vi "Command Select.vi"(8 "error in (no error)":errorcluster, 9 "Node Id":u8, 11 "Cmd Type":T1) -> (0 "error out":errorcluster, 2 "Cmd Str":string)   [LabVIEW 2011]
uses:
  Enumerator/CmdType.ctl
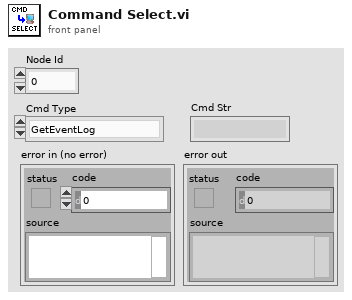
[diagram p1: front panel]
types:
  T1 = typedef "CmdType.ctl" = enum16{"GetEventLog", "DelTransaction", "InvalidMessage", "RelayControl", "RelayOff", "RelayOn", "VaildMessage", "EventPolling", "StoppingWaiting", "PromptKeying-in"}
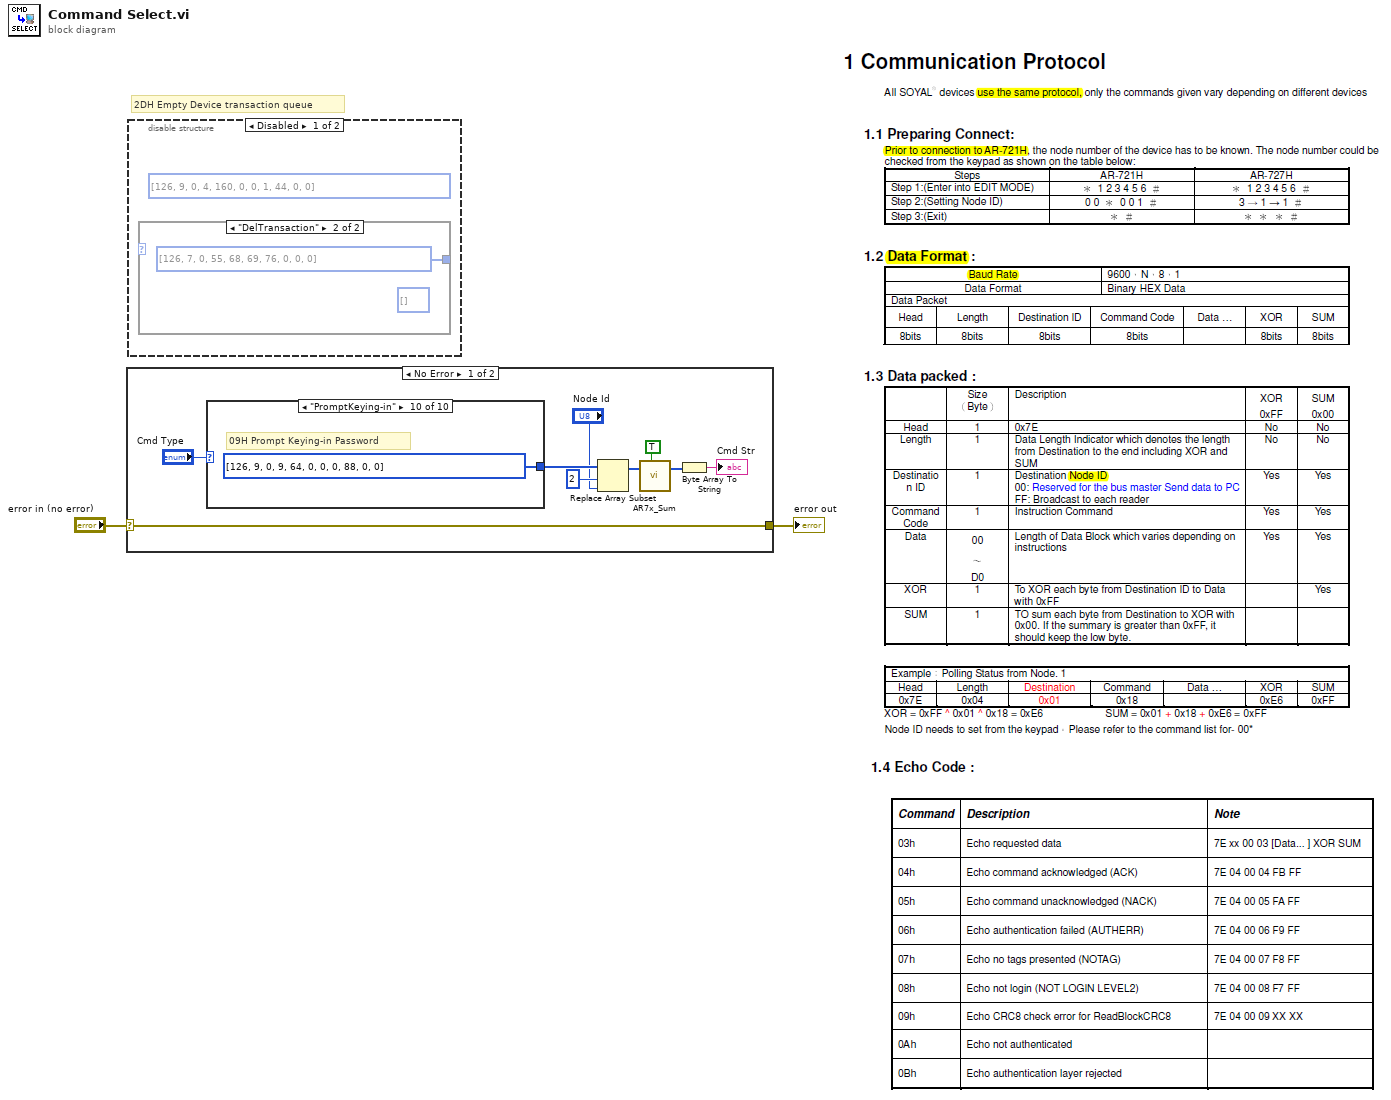
[diagram p0: block diagram]
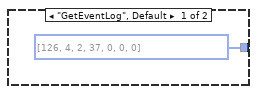
[diagram p2: hidden frame]
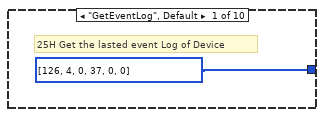
[diagram p4: hidden frame]
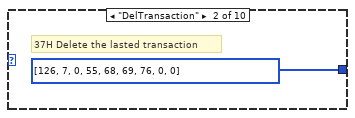
[diagram p5: hidden frame]
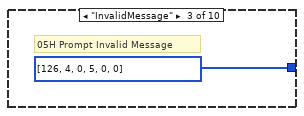
[diagram p6: hidden frame]
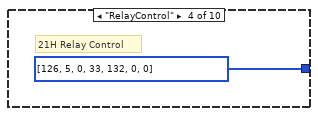
[diagram p7: hidden frame]
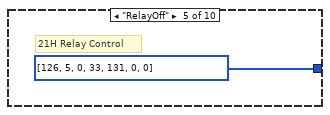
[diagram p8: hidden frame]
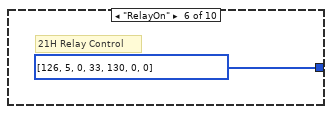
[diagram p9: hidden frame]
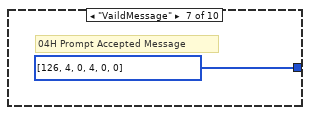
[diagram p10: hidden frame]
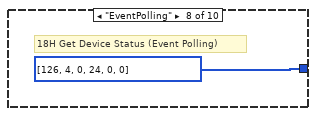
[diagram p11: hidden frame]
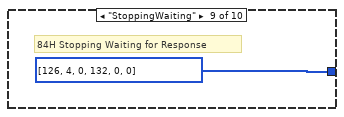
[diagram p12: hidden frame]
diagram:
  # "2DH Empty Device transaction queue"
  n1 = case shown="No Error" "error in (no error)" {
    selector: "error in (no error)" -> [w6 w22]
    tunnel: [w6 w22] -> w1
    frame No Error {
      n2 = case shown="\"PromptKeying-in\"" "Cmd Type" {
        tunnel: [u8[] [126, 4, 0, 37, 0, 0] u8[] [126, 7, 0, 55, 68, 69, 76, 0, 0] u8[] [126, 4, 0, 5, 0, 0] u8[] [126, 5, 0, 33, 132, 0, 0] u8[] [126, 5, 0, 33, 131, 0, 0] u8[] [126, 5, 0, 33, 130, 0, 0] u8[] [126, 4, 0, 4, 0, 0] u8[] [126, 4, 0, 24, 0, 0] u8[] [126, 4, 0, 132, 0, 0] u8[] [126, 9, 0, 9, 64, 0, 0, 0, 88, 0, 0]] -> w8
        frame "GetEventLog", Default {
          # "25H Get the lasted event Log of Device"
        }
        frame "DelTransaction" {
          # "37H Delete the lasted transaction"
        }
        frame "InvalidMessage" {
          # "05H Prompt Invalid Message"
        }
        frame "RelayControl" {
          # "21H Relay Control"
        }
        frame "RelayOff" {
          # "21H Relay Control"
        }
        frame "RelayOn" {
          # "21H Relay Control"
        }
        frame "VaildMessage" {
          # "04H Prompt Accepted Message"
        }
        frame "EventPolling" {
          # "18H Get Device Status (Event Polling)"
        }
        frame "StoppingWaiting" {
          # "84H Stopping Waiting for Response"
        }
        frame "PromptKeying-in" {
          # "09H Prompt Keying-in Password"
        }
      }
      n3 = Replace Array Subset(array=w8, new element="Node Id", index=2) -> (w9:u8[])
      n4 = call "AR7x_Sum.vi"("output"=TRUE, "Cmd In"=w9) -> ("Cmd Out"=w11:u8[])  [unwired: 6 in, 3 out]
      n5 = Byte Array To String(unsigned byte array=w11) -> (string=→"Cmd Str":string)
    }
    frame Error {
    }
  }
  "error out" <- w1
  n6 = disable-structure shown="Disabled" {
    frame Disabled {
      (unwired) u8[] [126, 9, 0, 4, 160, 0, 0, 1, 44, 0, 0]
      n7 = case shown="\"DelTransaction\"" {
        selector: _ -> [_ _]
        tunnel: [u8[] [126, 4, 2, 37, 0, 0, 0] u8[] [126, 7, 0, 55, 68, 69, 76, 0, 0, 0]] -> _
        frame "GetEventLog", Default {
        }
        frame "DelTransaction" {
          (unwired) u8[] []
        }
      }
    }
    frame Enabled {
    }
  }
